vi "instrument.vi"() -> ()   [LabVIEW 2016]
uses:
  <vilib>/Instr/_visa.llb/VISA Configure Serial Port (Instr).vi
panel:
  in  "Tab Control 3":enum32{"How to use ?", "Oscilloscope Commands"}(tab)
  out "number 4":dbl
  out "number 3":dbl
  out "read buffer 3":string
  out "Enum":enum16{"0", "1", "2", "3", "4", "5", "6", "7"}(ring)
  in  "Tab Control 2":enum32{"Commands", "Manual Command", "Settings"}(tab)
  in  "Set":bool
  in  "#Points":string
  in  "PLOT":bool
  in  "Measure 6":bool
  in  "Measure 5":bool
  in  "Measure 4":bool
  in  "Measure 3":bool
  in  "Measure 2":bool
  in  "Measure":bool
  out "RMS (V)":string
  out "PP (V)":string
  out "MAX (V)":string
  out "MIN (V)":string
  out "Average (V)":string
  out "Amplitude (V)":string
  in  "AUTOSCALE":bool
  in  "AUTOSCALE wrt.":T1(radio)
  in  "OK Button 4":bool
  in  "OK Button 3":bool
  in  "OK Button 2":bool
  in  "d ch1":bool
  out "read buffer 2":string
  out "return count 3":u32
  out "error out":errorcluster
  out "Waveform Graph":cluster{i32, dbl, dbl[]}(graph)
  in  "Read":bool
  in  "manual String 2":string
  in  "Write button 2":bool
  in  "VISA Open timeout (0)":u32
  in  "access mode":u32
  in  "VISA resource name 2":refnum<visa-resource-name>
  in  "duplicate session (F)":bool
  in  "Tab Control":T2(tab)
  in  "Get Errors":bool
  in  "System to Remote":bool
  in  "Clear":bool
  in  "Display":bool
  in  "Display Text":string
  in  "Apply":bool
  in  "Waveform":string(combo)
  in  "Offset (V)":string
  in  "Amplitude (V)":string
  in  "Frequency (Hz)":string
  out "read buffer":string
  out "return count 2":u32
  in  "Write button":bool
  in  "manual String":string
  out "return count":u32
  in  "VISA resource name":refnum<visa-resource-name>
  in  "timeout (10sec)":u32=10000
  in  "baud rate (9600)":u32=9600
  in  "data bits (8)":u16=8 min=5 max=8 step=1
  in  "parity (0:none)":enum16{"None", "Odd", "Even", "Mark", "Space"}(ring)
  in  "stop bits (10: 2 bit)":u16(ring)=20 items=["1.0"=10, "1.5"=15, "2.0"=20]
  in  "flow control (0:none)":u16(ring) items=["None", "XON/XOFF", "RTS/CTS", "XON/XOFF & RTS/CTS", "DTR/DSR", "XON/XOFF & DTR/DSR"]
  in  "Enable Termination\nChar (T)":bool=TRUE
  in  "termination char\n(0xA = '\\n' = LF)":u8=10 format="%.0x"
  # "Oscilloscope"
  # "Function Generator"
  # "How to Use ?\n\n-  Adjust the settings for ports in the settings tab\n- In manual command tabs, any command can send via serial link to the devices. To read the returning response check read button.\n- In function generator's command tab, waveforms with different shapes and properties can be created. A text can be set on the screen and the errors can be displayed.\n- In oscilloscope's command tab, different channels can be activated, different values can be measured, the plot on the screen can be autoscaled wrt. different channels. Lastly, first specifying the number of points that will be used on the graph, the graph on the screen of the oscilloscope can be displayed in the application."
  # "Commands used to communicate with oscilloscope\n\n:CHAN1:DISP 1 -> Open the display of channel 1\n:AUT CHAN1 -> Autoscale wrt. channel 1\n:MEAS:VAMP? -> Query the amplitude\n:MEAS:VAMP? -> Query the average voltage\n:MEAS:VMIN? -> Query the minumum voltage\n:MEAS:VMAX? -> Query the maximum voltage\n:MEAS:VPP? -> Query the peak-to-peak voltage\n:MEAS:VRMS? -> Query the rms voltage\n:WAV:DATA? -> Query waveform data, it returns in bytes form\n:WAV:POIN 1000 - > Get wav data with 1000 points\n:WAV:XINC?, :WAV:YINC? -> Query amount of increase in the graph per 1 y value\n:WAV:XREF?, :WAV:YREF? -> Query the position of the 0 voltage in the graph\n:MEAS:SOUR? -> Query channels for meauserements"
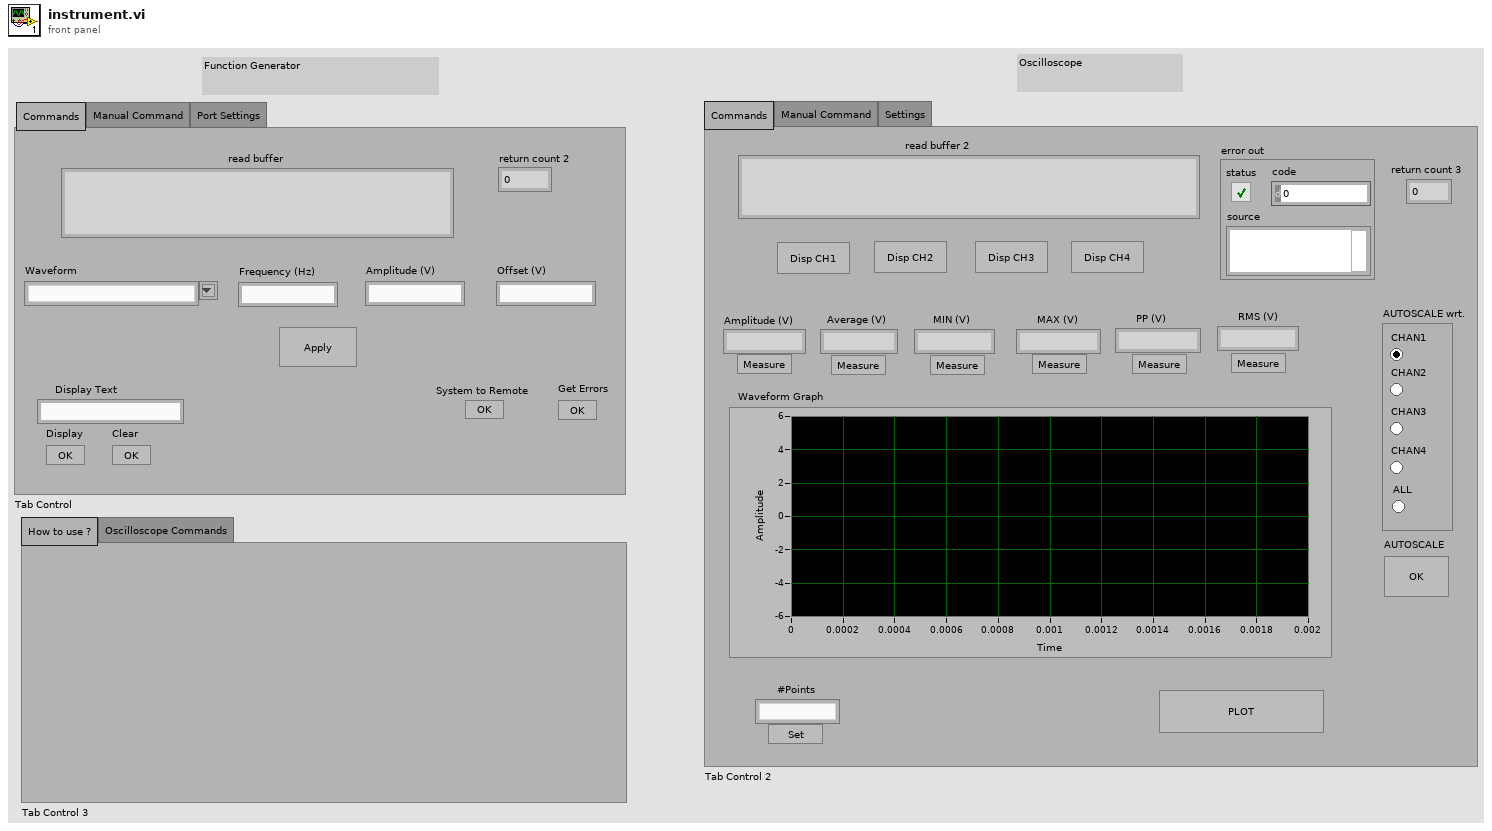
[diagram p1: front panel]
types:
  T1 = enum32{"CHAN1", "CHAN2", "CHAN3", "CHAN4", "ALL"}
  T2 = enum32{"Commands", "Manual Command", "Port Settings"}
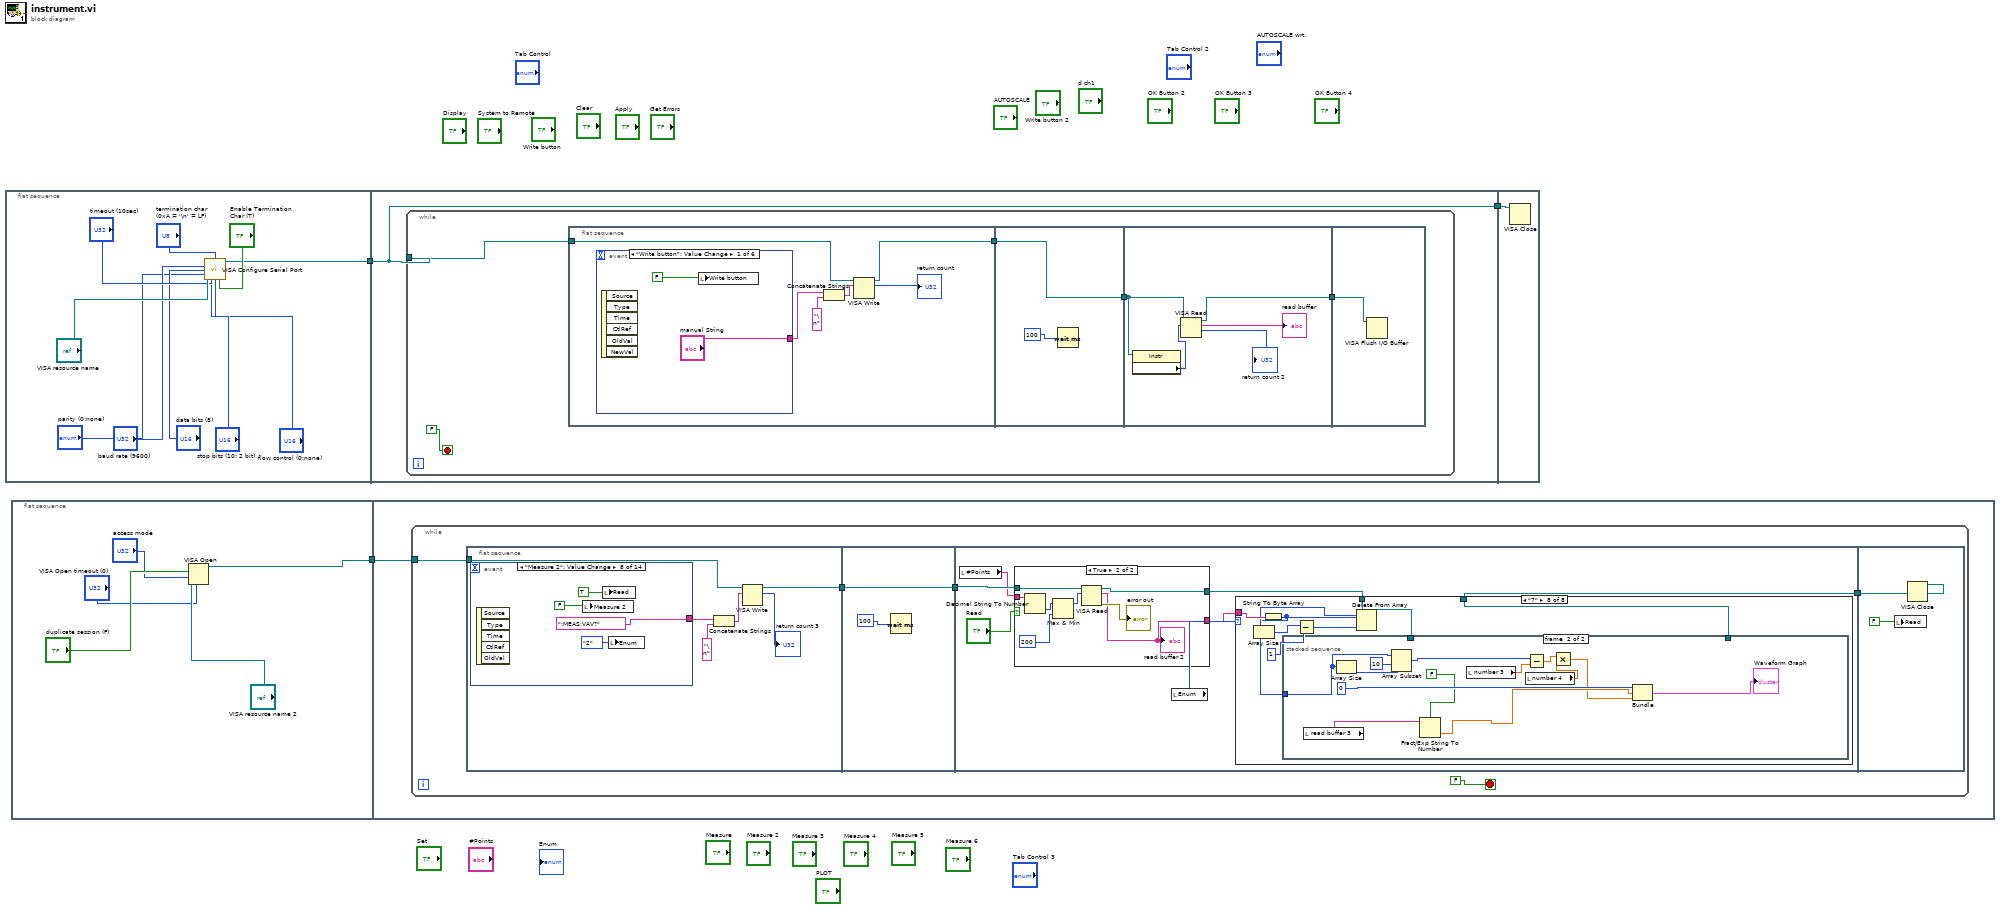
[diagram p0: block diagram]
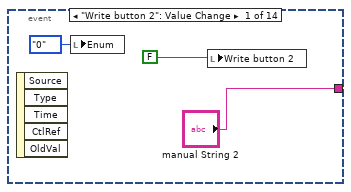
[diagram p2: hidden frame]
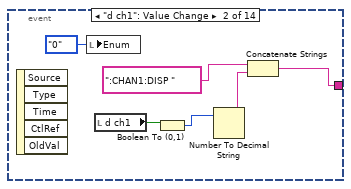
[diagram p3: hidden frame]
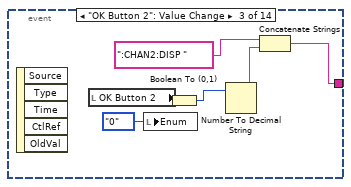
[diagram p4: hidden frame]
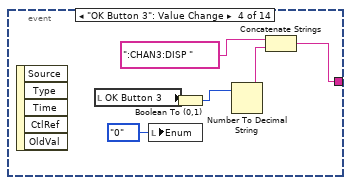
[diagram p5: hidden frame]
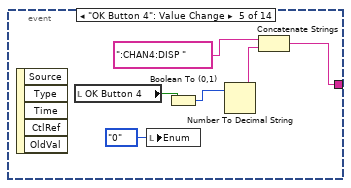
[diagram p6: hidden frame]
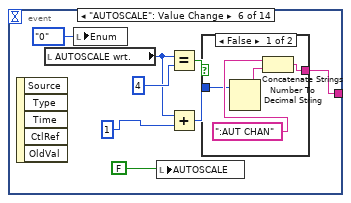
[diagram p7: hidden frame]
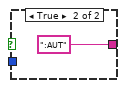
[diagram p8: hidden frame]
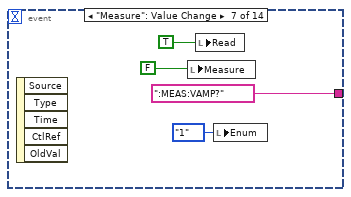
[diagram p9: hidden frame]
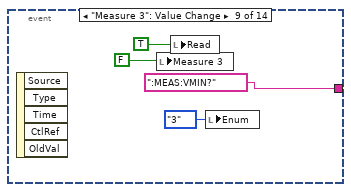
[diagram p10: hidden frame]
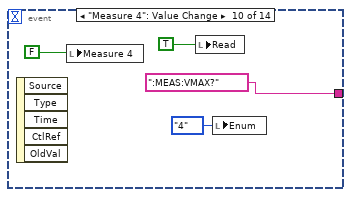
[diagram p11: hidden frame]
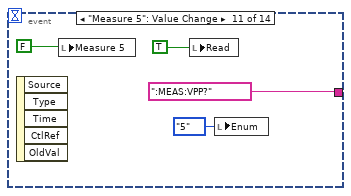
[diagram p12: hidden frame]
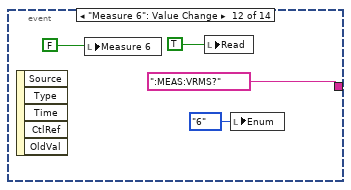
[diagram p13: hidden frame]
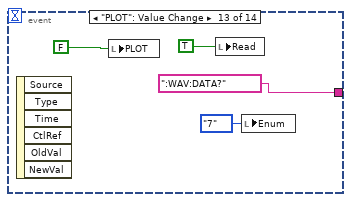
[diagram p14: hidden frame]
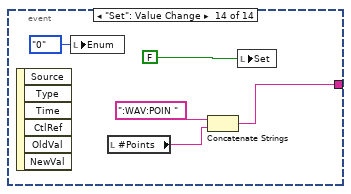
[diagram p15: hidden frame]
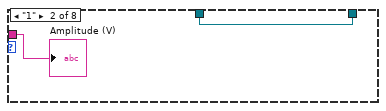
[diagram p17: hidden frame]
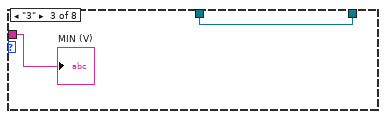
[diagram p18: hidden frame]
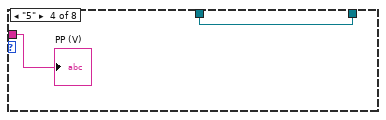
[diagram p19: hidden frame]
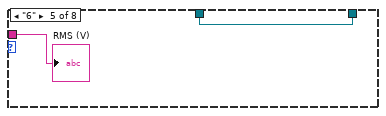
[diagram p20: hidden frame]
diagram:
  n1 = flat-sequence {
    tunnel: [w4] -> w3
    tunnel: w3 -> [w14]
    tunnel: [w14] -> w2
    tunnel: w2 -> [w55]
    frame #0 {
      n2 = call-poly "VISA Configure Serial Port"("VISA resource name"="VISA resource name", "timeout (10sec)"="timeout (10sec)", "termination char\n(0xA = '\\n' = LF)"="termination char\n(0xA = '\\n' = LF)", "Enable Termination\nChar (T)"="Enable Termination\nChar (T)", "baud rate (9600)"="baud rate (9600)", "data bits (8)"="data bits (8)", "parity (0:none)"="parity (0:none)", "stop bits (10: 1 bit)"="stop bits (10: 2 bit)", "flow control (0:none)"="flow control (0:none)") -> ("VISA resource name out"=w4:refnum<visa-resource-name>)  [unwired: 5 in, 1 out]
    }
    frame #1 {
      n3 = while {
        tunnel: w14 -> [w19]
        stop <- FALSE stop-if-true
        n4 = flat-sequence {
          tunnel: w19 -> [w25]
          tunnel: [w24] -> w18
          tunnel: [w48] -> w17
          tunnel: w18 -> [w48]
          tunnel: [w49] -> w16
          tunnel: w17 -> [w50]
          tunnel: w16 -> [w54]
          frame #0 {
            n5 = event shown="[0] \"Write button\": Value Change" {
              selector: _ -> [_ _ _ _ _ _]
              dyn-events: _ -> [_ _ _ _ _ _]
              timeout: _ -> [_ _ _ _ _ _]
              tunnel: ["manual String" w32 "SYST:ERR?" "SYST:REM" w43 "DISP:TEXT:CLE"] -> w22
              event "Write button": Value Change {
                n6 = event-data() -> ()  [unwired: 1 in, 6 out]
                n7 = local write "Write button"(FALSE) -> ()
              }
              event "Apply": Value Change {
                n8 = event-data() -> ()  [unwired: 1 in, 6 out]
                n9 = local write "Apply"(FALSE) -> ()
                n10 = Format Into String(format string="%s%s %s, %s, %s", "APPL:", "Waveform", "Frequency (Hz)", "Amplitude (V)", "Offset (V)") -> (resulting string=w32:string)  [unwired: 2 in, 1 out]
              }
              event "Get Errors": Value Change {
                n11 = event-data() -> ()  [unwired: 1 in, 6 out]
                n12 = local write "Get Errors"(FALSE ("Get Errors")) -> ()
              }
              event "System to Remote": Value Change {
                n13 = event-data() -> ()  [unwired: 1 in, 6 out]
                n14 = local write "System to Remote"(FALSE) -> ()
              }
              event "Display": Value Change {
                n15 = event-data() -> ()  [unwired: 1 in, 6 out]
                n16 = local write "Display"(FALSE ("Display")) -> ()
                n17 = Format Into String(format string="%s\"%s\"", "DISP:TEXT ", "Display Text") -> (resulting string=w43:string)  [unwired: 2 in, 1 out]
              }
              event "Clear": Value Change {
                n18 = event-data() -> ()  [unwired: 1 in, 6 out]
                n19 = local write "Clear"(FALSE ("Clear")) -> ()
              }
            }
            n20 = Concatenate Strings(w22, "\n") -> (w21:string)
            n21 = VISA Write(VISA resource name=w25, write buffer=w21) -> (VISA resource name out=w24:refnum<visa-resource-name>, return count=→"return count":u32)  [unwired: 1 in, 1 out]
          }
          frame #1 {
            n22 = Wait (ms)(milliseconds to wait=u32 100 ("millisecond timer value")) -> ()  [unwired: 1 out]
          }
          frame #2 {
            n23 = property class="Instr"(reference=w50) -> ("Serial Settings:Number of Bytes at Serial Port"=w51:u32)  [unwired: 1 in, 2 out]
            n24 = VISA Read(VISA resource name=w50, byte count=w51) -> (VISA resource name out=w49:refnum<visa-resource-name>, read buffer=→"read buffer":string, return count=→"return count 2":u32)  [unwired: 1 in, 1 out]
          }
          frame #3 {
            n25 = VISA Flush I/O Buffer(VISA resource name=w54) -> ()  [unwired: 2 in, 2 out]
          }
        }
      }
    }
    frame #2 {
      n26 = VISA Close(VISA resource name=w55) -> ()  [unwired: 1 in, 1 out]
    }
  }
  n27 = flat-sequence {
    tunnel: [w56] -> w1
    tunnel: w1 -> [w61]
    frame #0 {
      n28 = VISA Open(timeout (0)="VISA Open timeout (0)", duplicate session (F)="duplicate session (F)", access mode="access mode", VISA resource name="VISA resource name 2") -> (VISA resource name=w56:refnum<visa-resource-name>)  [unwired: 1 in, 1 out]
    }
    frame #1 {
      n29 = while {
        tunnel: w61 -> [w66]
        stop <- FALSE stop-if-true
        n30 = flat-sequence {
          tunnel: w66 -> [w70]
          tunnel: [w67] -> w64
          tunnel: [w147] -> w65
          tunnel: w64 -> [w147]
          tunnel: w65 -> [w154]
          tunnel: [w148] -> w63
          tunnel: w63 -> [w223]
          frame #0 {
            n31 = event shown="[7] \"Measure 2\": Value Change" {
              selector: _ -> [_ _ _ _ _ _ _ _ _ _ _ _ _ _]
              dyn-events: _ -> [_ _ _ _ _ _ _ _ _ _ _ _ _ _]
              timeout: _ -> [_ _ _ _ _ _ _ _ _ _ _ _ _ _]
              tunnel: ["manual String 2" w77 w83 w89 w95 w106 ":MEAS:VAMP?" ":MEAS:VAV?" ":MEAS:VMIN?" ":MEAS:VMAX?" ":MEAS:VPP?" ":MEAS:VRMS?" ":WAV:DATA?" w141] -> w71
              event "Write button 2": Value Change {
                n32 = event-data() -> ()  [unwired: 1 in, 5 out]
                n33 = local write "Enum"(enum16{"0", "1", "2", "3", "4", "5", "6"}."0" ("Enum")) -> ()
                n34 = local write "Write button 2"(FALSE) -> ()
              }
              event "d ch1": Value Change {
                n35 = event-data() -> ()  [unwired: 1 in, 5 out]
                n36 = local write "Enum"(enum16{"0", "1", "2", "3", "4", "5", "6"}."0" ("Enum")) -> ()
                n37 = local read "d ch1"() -> (w81:bool)
                n38 = Boolean To (0,1)(Boolean=w81) -> (0, 1=w80:i16)
                n39 = Number To Decimal String(number=w80) -> (decimal integer string=w78:string)  [unwired: 1 in]
                n40 = Concatenate Strings(":CHAN1:DISP ", w78) -> (w77:string)
              }
              event "OK Button 2": Value Change {
                n41 = event-data() -> ()  [unwired: 1 in, 5 out]
                n42 = local read "OK Button 2"() -> (w87:bool)
                n43 = local write "Enum"(enum16{"0", "1", "2", "3", "4", "5", "6"}."0" ("Enum")) -> ()
                n44 = Boolean To (0,1)(Boolean=w87) -> (0, 1=w86:i16)
                n45 = Number To Decimal String(number=w86) -> (decimal integer string=w84:string)  [unwired: 1 in]
                n46 = Concatenate Strings(":CHAN2:DISP ", w84) -> (w83:string)
              }
              event "OK Button 3": Value Change {
                n47 = event-data() -> ()  [unwired: 1 in, 5 out]
                n48 = local read "OK Button 3"() -> (w93:bool)
                n49 = local write "Enum"(enum16{"0", "1", "2", "3", "4", "5", "6"}."0" ("Enum")) -> ()
                n50 = Boolean To (0,1)(Boolean=w93) -> (0, 1=w92:i16)
                n51 = Number To Decimal String(number=w92) -> (decimal integer string=w90:string)  [unwired: 1 in]
                n52 = Concatenate Strings(":CHAN3:DISP ", w90) -> (w89:string)
              }
              event "OK Button 4": Value Change {
                n53 = event-data() -> ()  [unwired: 1 in, 5 out]
                n54 = local read "OK Button 4"() -> (w99:bool)
                n55 = local write "Enum"(enum16{"0", "1", "2", "3", "4", "5", "6"}."0" ("Enum")) -> ()
                n56 = Boolean To (0,1)(Boolean=w99) -> (0, 1=w98:i16)
                n57 = Number To Decimal String(number=w98) -> (decimal integer string=w96:string)  [unwired: 1 in]
                n58 = Concatenate Strings(":CHAN4:DISP ", w96) -> (w95:string)
              }
              event "AUTOSCALE": Value Change {
                n59 = event-data() -> ()  [unwired: 1 in, 5 out]
                n60 = local read "AUTOSCALE wrt."() -> (w104:T1)
                n61 = local write "Enum"(enum16{"0", "1", "2", "3", "4", "5", "6"}."0" ("Enum")) -> ()
                n62 = local write "AUTOSCALE"(FALSE) -> ()
                n63 = Equal?(x=w104, y=4) -> (x = y?=w107:bool)
                n64 = Add(x=w104, y=1) -> (x+y=w102:u32)
                n65 = case shown="False" w107 {
                  tunnel: [w109 ":AUT"] -> w106
                  tunnel: w102 -> [w108 _]
                  frame False {
                    n66 = Number To Decimal String(number=w108) -> (decimal integer string=w110:string)  [unwired: 1 in]
                    n67 = Concatenate Strings(":AUT CHAN", w110) -> (w109:string)
                  }
                  frame True {
                  }
                }
              }
              event "Measure": Value Change {
                n68 = event-data() -> ()  [unwired: 1 in, 5 out]
                n69 = local write "Measure"(FALSE) -> ()
                n70 = local write "Read"(TRUE ("Read Also")) -> ()
                n71 = local write "Enum"(enum16{"0", "1", "2", "3", "4", "5", "6"}."1" ("Enum")) -> ()
              }
              event "Measure 2": Value Change {
                n72 = event-data() -> ()  [unwired: 1 in, 5 out]
                n73 = local write "Measure 2"(FALSE) -> ()
                n74 = local write "Read"(TRUE ("Read Also")) -> ()
                n75 = local write "Enum"(enum16{"0", "1", "2", "3", "4", "5", "6"}."2" ("Enum")) -> ()
              }
              event "Measure 3": Value Change {
                n76 = event-data() -> ()  [unwired: 1 in, 5 out]
                n77 = local write "Measure 3"(FALSE) -> ()
                n78 = local write "Read"(TRUE ("Read Also")) -> ()
                n79 = local write "Enum"(enum16{"0", "1", "2", "3", "4", "5", "6"}."3" ("Enum")) -> ()
              }
              event "Measure 4": Value Change {
                n80 = event-data() -> ()  [unwired: 1 in, 5 out]
                n81 = local write "Measure 4"(FALSE) -> ()
                n82 = local write "Read"(TRUE ("Read Also")) -> ()
                n83 = local write "Enum"(enum16{"0", "1", "2", "3", "4", "5", "6"}."4" ("Enum")) -> ()
              }
              event "Measure 5": Value Change {
                n84 = event-data() -> ()  [unwired: 1 in, 5 out]
                n85 = local write "Measure 5"(FALSE) -> ()
                n86 = local write "Read"(TRUE ("Read Also")) -> ()
                n87 = local write "Enum"(enum16{"0", "1", "2", "3", "4", "5", "6"}."5" ("Enum")) -> ()
              }
              event "Measure 6": Value Change {
                n88 = event-data() -> ()  [unwired: 1 in, 5 out]
                n89 = local write "Measure 6"(FALSE) -> ()
                n90 = local write "Read"(TRUE ("Read Also")) -> ()
                n91 = local write "Enum"(enum16{"0", "1", "2", "3", "4", "5", "6"}."6" ("Enum")) -> ()
              }
              event "PLOT": Value Change {
                n92 = event-data() -> ()  [unwired: 1 in, 6 out]
                n93 = local write "PLOT"(FALSE) -> ()
                n94 = local write "Read"(TRUE ("Read Also")) -> ()
                n95 = local write "Enum"(enum16{"0", "1", "2", "3", "4", "5", "6", "7"}."7" ("Enum")) -> ()
              }
              event "Set": Value Change {
                n96 = event-data() -> ()  [unwired: 1 in, 6 out]
                n97 = local write "Enum"(enum16{"0", "1", "2", "3", "4", "5", "6"}."0" ("Enum")) -> ()
                n98 = local read "#Points"() -> (w142:string)
                n99 = Concatenate Strings(":WAV:POIN ", w142) -> (w141:string)
                n100 = local write "Set"(FALSE) -> ()
              }
            }
            n101 = Concatenate Strings(w71, "\n") -> (w69:string)
            n102 = VISA Write(VISA resource name=w70, write buffer=w69) -> (VISA resource name out=w67:refnum<visa-resource-name>, return count=→"return count 3":u32)  [unwired: 1 in, 1 out]
          }
          frame #1 {
            n103 = Wait (ms)(milliseconds to wait=u32 100 ("millisecond timer value")) -> ()  [unwired: 1 out]
          }
          frame #2 {
            n104 = local read "#Points"() -> (w150:string)
            n105 = case shown="True" "Read" {
              tunnel: w154 -> [w213 w221]
              tunnel: [w213 w220] -> w149
              tunnel: ["" w218] -> w151
              tunnel: w150 -> [_ w215]
              frame False {
              }
              frame True {
                n106 = Decimal String To Number(string=w215) -> (number=w214:i32)  [unwired: 2 in, 1 out]
                n107 = Max & Min(x=w214, y=200) -> (max(x,y)=w216:i32)  [unwired: 1 out]
                n108 = VISA Read(VISA resource name=w221, byte count=w216) -> (VISA resource name out=w220:refnum<visa-resource-name>, read buffer=w218:string, error out=→"error out":errorcluster)  [unwired: 1 in, 1 out]
                "read buffer 2" <- w218
              }
            }
            n109 = local read "Enum"() -> (w152:enum16{"0", "1", "2", "3", "4", "5", "6", "7"})
            n110 = case shown="\"7\"" w152 {
              tunnel: w151 -> [_ w157 w159 w161 w163 w165 w167 w175]
              tunnel: w149 -> [w155 w156 w158 w160 w162 w164 w166 w174]
              tunnel: [w155 w156 w158 w160 w162 w164 w166 w168] -> w148
              frame "0", Default {
              }
              frame "1" {
                "Amplitude (V)" <- w157
              }
              frame "3" {
                "MIN (V)" <- w159
              }
              frame "5" {
                "PP (V)" <- w161
              }
              frame "6" {
                "RMS (V)" <- w163
              }
              frame "4" {
                "MAX (V)" <- w165
              }
              frame "2" {
                "Average (V)" <- w167
              }
              frame "7" {
                n111 = String To Byte Array(string=w175) -> (unsigned byte array=w172:u8[])
                n112 = Array Size(array=w172) -> (size(s)=w171:i32)
                n113 = Subtract(x=w171, y=1) -> (x-y=w170:i32)
                n114 = Delete From Array(array=w172, index=w170) -> (array with subset deleted=w173:u8[])  [unwired: 1 in, 1 out]
                n115 = stacked-sequence {
                  tunnel: w173 -> [_ w209]
                  tunnel: w174 -> [w197 _]
                  tunnel: [w183 _] -> w168
                  frame #0 {
                    n116 = VISA Write(VISA resource name=w197, write buffer=":WAV:XINC?\n") -> (VISA resource name out=w195:refnum<visa-resource-name>, error out=w189:errorcluster)  [unwired: 1 in, 1 out]
                    n117 = local write "error out"(w189) -> ()
                    n118 = VISA Read(VISA resource name=w195, byte count=u32 100) -> (VISA resource name out=w190:refnum<visa-resource-name>, read buffer=→"read buffer 3":string)  [unwired: 1 in, 2 out]
                    n119 = VISA Write(VISA resource name=w190, write buffer=":WAV:YREF?\n") -> (VISA resource name out=w193:refnum<visa-resource-name>, error out=w188:errorcluster)  [unwired: 1 in, 1 out]
                    n120 = local write "error out"(w188) -> ()
                    n121 = VISA Read(VISA resource name=w193, byte count=u32 100) -> (VISA resource name out=w184:refnum<visa-resource-name>, read buffer=w181:string)  [unwired: 1 in, 2 out]
                    n122 = Fract/Exp String To Number(use system decimal point (T)=FALSE ("use system decimal point (T) 2"), string=w181) -> (number=→"number 3":dbl)  [unwired: 2 in, 1 out]
                    n123 = VISA Write(VISA resource name=w184, write buffer=":WAV:YINC?\n") -> (VISA resource name out=w185:refnum<visa-resource-name>, error out=w187:errorcluster)  [unwired: 1 in, 1 out]
                    n124 = local write "error out"(w187) -> ()
                    n125 = VISA Read(VISA resource name=w185, byte count=u32 100) -> (VISA resource name out=w183:refnum<visa-resource-name>, read buffer=w179:string)  [unwired: 1 in, 2 out]
                    n126 = Fract/Exp String To Number(use system decimal point (T)=FALSE ("use system decimal point (T) 2"), string=w179) -> (number=→"number 4":dbl)  [unwired: 2 in, 1 out]
                  }
                  frame #1 {
                    n127 = local read "read buffer 3"() -> (w207:string)
                    n128 = Array Size(array=w209) -> (size(s)=w210:i32)
                    n129 = Array Subset(array=w209, index=10, length=w210) -> (w203:u8[])
                    n130 = Fract/Exp String To Number(use system decimal point (T)=FALSE ("use system decimal point (T) 2"), string=w207) -> (number=w205:dbl)  [unwired: 2 in, 1 out]
                    n131 = local read "number 3"() -> (w204:dbl)
                    n132 = local read "number 4"() -> (w200:dbl)
                    n133 = Subtract(x=w203, y=w204) -> (x-y=w201:dbl[])
                    n134 = Multiply(x=w201, y=w200) -> (x*y=w202:dbl[])
                    n135 = Bundle(0, w205, w202) -> (→"Waveform Graph":cluster{i32, dbl, dbl[]})  [unwired: 1 in]
                  }
                }
              }
            }
          }
          frame #3 {
            n136 = local write "Read"(FALSE ("Read Also")) -> ()
            n137 = VISA Close(VISA resource name=w223) -> ()  [unwired: 1 in, 1 out]
          }
        }
      }
    }
  }
